vi "Check for Transceiver Errors.vi"(8 "error in (no error)":errorcluster, 11 "Framework in":refnum<class "Framework.lvclass">) -> (0 "error out":errorcluster, 3 "Framework out":refnum<class "Framework.lvclass">)   [LabVIEW 2017, in "DSF Core.lvlib" / "Framework.lvclass"]
uses:
  Framework.lvclass
  Framework.lvclass/Framework.ctl
  Plugin/Plugin.lvclass/Plugin.ctl
  Interfaces/Interface/Interface.lvclass/Interface.ctl
  Interfaces/Interface/Errors.ctl
  Interfaces/Transceiver Interface/Read Plugin Error.vi
  Interfaces/Interface/Read Error.vi
  Interfaces/Interface/Read Error Queue.vi
  Interfaces/Transceiver Interface/Plugin Interface.lvclass
  C:/Users/Admin/Desktop/Data Sharing Framework/Source/Core/Engine/Classes/Interfaces/Interface/Interface.lvclass
  Interfaces/Interface/Errors.vi
  Interfaces/Dispatcher/Error Timeout.vi
  Interfaces/Transceiver Interface/Class Name.vi
  Plugin/Plugin.lvclass
  Interfaces/Interface/Interface.lvclass
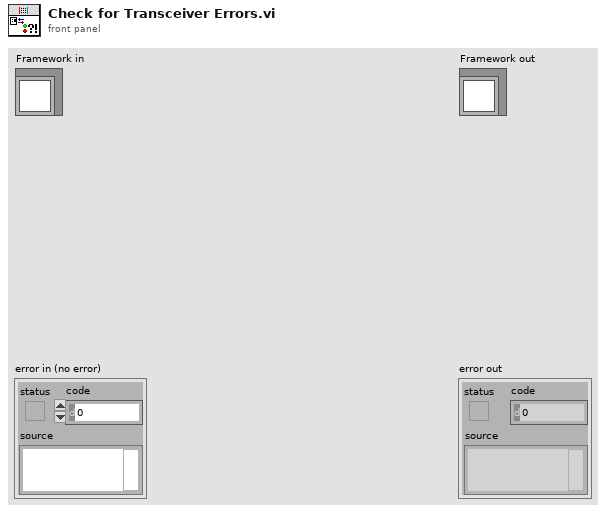
[diagram p1: front panel]
types:
  T1 = typedef "DSF Core.lvlib/Interface.lvclass/Errors.ctl" = enum16{"Command Timeout", "Response Timeout", "Error Timeout", "Invalid Response", "Invalid Response Parameters"}
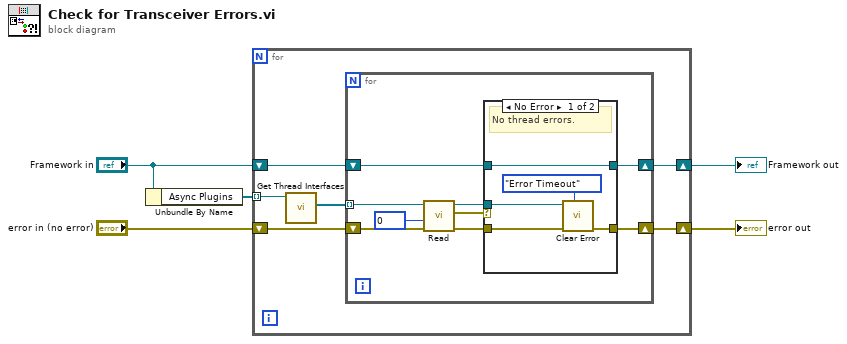
[diagram p0: block diagram]
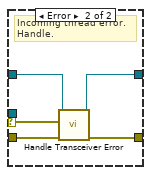
[diagram p2: hidden frame]
diagram:
  n1 = Unbundle By Name("Framework in") -> ("Async Plugins"=w3:refnum<class "Plugin.lvclass">[])
  n2 = for {
    tunnel: w3 -> [w11] mode=indexing
    shift-right: [w8] -> w4
    shift-left: "error in (no error)" -> [w9]
    shift-right: [w6] -> w1
    shift-left: "Framework in" -> [w7]
    n3 = call "Get Thread Interfaces.vi"("Plugin in"=w11) -> ("Plugin Interfaces"=w10:refnum<class "Plugin Interface.lvclass">[])  [unwired: 9 in, 1 out]
    n4 = for {
      tunnel: w10 -> [w20] mode=indexing
      shift-right: [w17] -> w8
      shift-left: w9 -> [w19]
      shift-right: [w15] -> w6
      shift-left: w7 -> [w16]
      n5 = call-poly "Read.vi"("error in (no error)"=w19, "timeout in ms (0)"=0, "Plugin Interface in"=w20) -> ("error out"=w14:errorcluster, "error"=w13:errorcluster, "Plugin Interface out"=w12:refnum<class "Plugin Interface.lvclass">)  [unwired: 6 in]
      n6 = case shown="No Error" w13 {
        selector: w13 -> [_ w26]
        tunnel: w14 -> [w24 w28]
        tunnel: [w23 w27] -> w17
        tunnel: w16 -> [w25 w30]
        tunnel: [w25 w29] -> w15
        tunnel: w12 -> [w22 _]
        frame No Error {
          # "No thread errors."
          n7 = call "Clear Error.vi"("error to clear"=Errors."Error Timeout", "error in (no error)"=w24, "Interface in"=w22) -> ("error out"=w23:errorcluster)  [unwired: 7 in, 1 out]
        }
        frame Error {
          # "Incoming thread error. Handle."
          n8 = call "Handle Transceiver Error.vi"("error in (no error)"=w28, "transceiver error"=w26, "Framework in"=w30) -> ("error out"=w27:errorcluster, "Framework out"=w29:refnum<class "Framework.lvclass">)  [unwired: 7 in]
        }
      }
    }
  }
  "error out" <- w4
  "Framework out" <- w1
